vi "gettingtowater.vi"() -> ()   [LabVIEW 2020]
uses:
  common/record_file_handler/VFH-VNA_File_Handler.lvlib
panel:
  out "Z Modulus":cluster{"Frequency":dbl[], "Array":dbl[]}
  out "Epsilon":cluster{"Array":dbl[], "Array":dbl[]}
  in  "Folder Path":path=path "C:/NanoVNA-App/Recordings/2024-07-26 09-29-22"
  out "Calc":cluster{"Frequency":dbl[], "S11_Imag":dbl[]}[](graph)
  out "Raw":cluster{"Frequency":dbl[], "S21_Imag":dbl[]}[](graph)
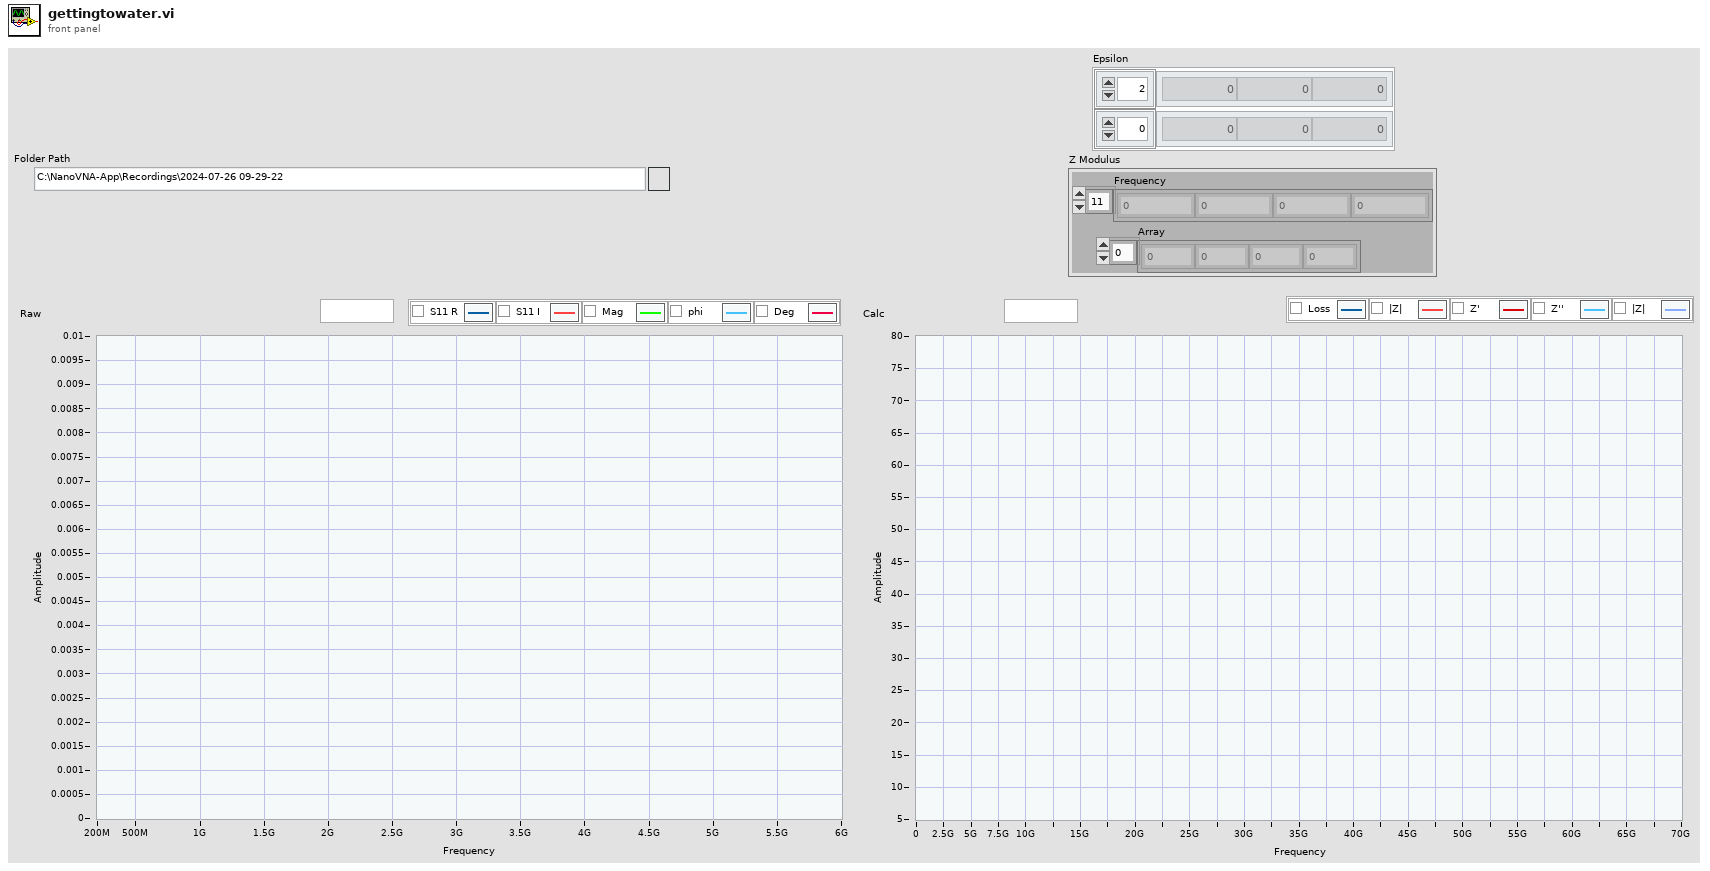
[diagram p1: front panel]
types:
  T1 = typedef "VFH-VNA_File_Handler.lvlib/VFH-file_cluster-NanoVNA.ctl" = cluster{"Frequency":dbl[], "S11_Real":dbl[], "S11_Imag":dbl[], "S21_Real":dbl[], "S21_Imag":dbl[], "S12_Real":dbl[], "S12_Imag":dbl[], "S22_Real":dbl[], "S22_Imag":dbl[]}
  T2 = cluster{"Loss":cluster{"Frequency":dbl[], "Array":dbl[]}, "Z Modulus":cluster{"Frequency":dbl[], "Array":dbl[]}, "Z'":cluster{"Frequency":dbl[], "Array":dbl[]}, "Z''":cluster{"Frequency":dbl[], "Array":dbl[]}}
  T3 = cluster{"S11'":cluster{"Frequency":dbl[], "S11_Real":dbl[]}, "S11''":cluster{"Frequency":dbl[], "S11_Real":dbl[]}, "Magnitude":cluster{"Frequency":dbl[], "Array":dbl[]}, "Eta":cluster{"Frequency":dbl[], "Array":dbl[]}, "Phase":cluster{"Frequency":dbl[], "Array":dbl[]}}
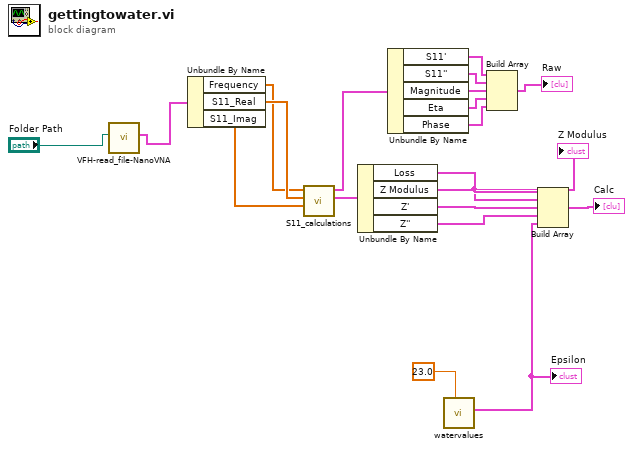
[diagram p0: block diagram]
diagram:
  n1 = call "VFH-read_file-NanoVNA.vi"("file path (dialog if empty)"="Folder Path") -> ("output cluster"=w7:T1)  [unwired: 9 in, 1 out]
  n2 = Unbundle By Name(w7) -> ("Frequency"=w3:dbl[], "S11_Real"=w5:dbl[], "S11_Imag"=w4:dbl[])
  n3 = call "S11_calculations.vi"("S11_Imag"=w4, "S11_Real"=w5, "Frequency"=w3) -> ("Calc"=w13:T2, "Raw"=w19:T3)  [unwired: 6 in, 1 out]
  n4 = Unbundle By Name(w13) -> ("Loss"=w12:cluster{"Frequency":dbl[], "Array":dbl[]}, "Z Modulus"=w2:cluster{"Frequency":dbl[], "Array":dbl[]}, "Z'"=w11:cluster{"Frequency":dbl[], "Array":dbl[]}, "Z''"=w10:cluster{"Frequency":dbl[], "Array":dbl[]})
  "Z Modulus" <- w2
  n5 = Unbundle By Name(w19) -> ("S11'"=w18:cluster{"Frequency":dbl[], "S11_Real":dbl[]}, "S11''"=w17:cluster{"Frequency":dbl[], "S11_Real":dbl[]}, "Magnitude"=w16:cluster{"Frequency":dbl[], "Array":dbl[]}, "Eta"=w15:cluster{"Frequency":dbl[], "Array":dbl[]}, "Phase"=w14:cluster{"Frequency":dbl[], "Array":dbl[]})
  n6 = call "watervalues.vi"("deg"=23.0) -> ("Epsilon"=w1:cluster{"Array":dbl[], "Array":dbl[]})  [unwired: 9 in, 1 out]
  "Epsilon" <- w1
  n7 = Build Array(w18, w17, w16, w15, w14) -> (→"Raw":cluster{"Frequency":dbl[], "Array":dbl[]}[])
  n8 = Build Array(w12, w2, w11, w10, w1) -> (→"Calc":cluster{"Array":dbl[], "Array":dbl[]}[])
